vi "Get Derivative Gain.vi"(4 "error in (no error)":errorcluster, 6 "Axis (1)":i32=1 min=1 max=3, 7 "VISA resource name":refnum<visa-resource-name>) -> (0 "error out":errorcluster, 2 "Kd":dbl format="%.4g", 3 "VISA resource name out":refnum<visa-resource-name>)   [LabVIEW 2012, in "Newport ESP301.lvlib"]
doc: "Reads the derivative gain factor Kd of the PID closed loop."
uses:
  Newport ESP301.lvlib
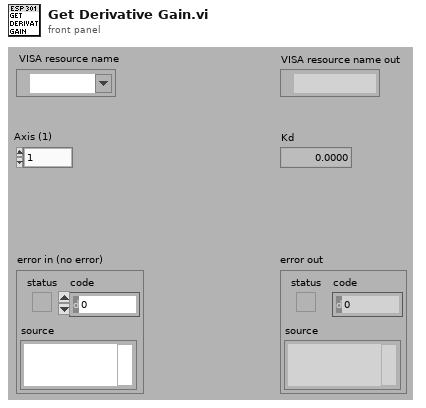
[diagram p1: front panel]
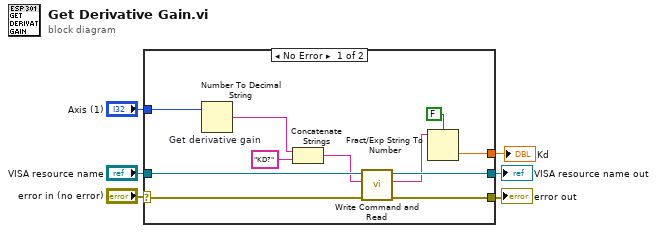
[diagram p0: block diagram]
diagram:
  n1 = case shown="No Error" "error in (no error)" {
    selector: "error in (no error)" -> [w14 w19]
    tunnel: [w16 w19] -> w6
    tunnel: "VISA resource name" -> [w17 w18]
    tunnel: [w15 w18] -> w5
    tunnel: "Axis (1)" -> [w13 _]
    tunnel: [w9 _] -> w1
    frame No Error {
      w12 = "KD?"  # Get derivative gain
      n2 = Number To Decimal String(number=w13) -> (decimal integer string=w11:string)  [unwired: 1 in]
      n3 = Concatenate Strings(w11, w12) -> (w10:string)
      n4 = call "Write Command and Read.vi"("error in (no error)"=w14, "Command"=w10, "VISA resource name"=w17) -> ("error out"=w16:errorcluster, "Returned string"=w8:string, "VISA resource name out"=w15:refnum<visa-resource-name>)  [unwired: 4 in]
      n5 = Fract/Exp String To Number(use system decimal point (T)=FALSE ("utiliser le séparateur décimal du système (V)"), string=w8) -> (number=w9:dbl)  [unwired: 2 in, 1 out]
    }
    frame Error {
    }
  }
  "error out" <- w6
  "VISA resource name out" <- w5
  "Kd" <- w1
